vi "Init.vi"(10 "Queue jettl":refnum<class "Queue jettl.lvclass">) -> (3 "Queue Last Ack Msg Strategy out":refnum<class "Queue Last Ack Msg Strategy.lvclass">)   [LabVIEW 2021, in "jettl.lvlib" / "Queue Last Ack.lvlib" / "Queue Last Ack Msg Strategy.lvclass"]
uses:
  Queue Last Ack Msg Strategy.lvclass
  Queue jettl/Queue jettl.lvclass
  Queue Last Ack Msg Strategy.lvclass/Queue Last Ack Msg Strategy.ctl
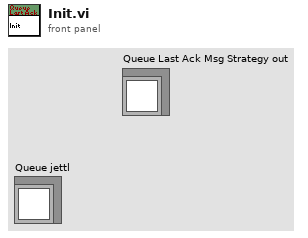
[diagram p1: front panel]
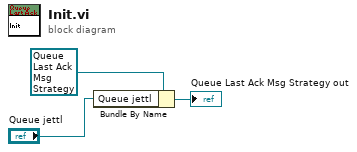
[diagram p0: block diagram]
diagram:
  n1 = Bundle By Name(cluster=refnum<class "Queue Last Ack Msg Strategy.lvclass"> refnum ("Last Ack Msg in"), "Queue jettl"="Queue jettl") -> (→"Queue Last Ack Msg Strategy out":refnum<class "Queue Last Ack Msg Strategy.lvclass">)
